vi "dvp Vi Set Target Format.vi"(10 "TargetFormat":u32(ring) items=["S_RAW8"=0, "S_RAW10"=1, "S_RAW12"=2, "S_RAW14"=3, "S_RAW16"=4, "S_BGR24"=10, "S_YCBCR_411"=20, "S_YCBCR_422"=21, "S_YCBCR_444"=22, "S_MONO8"=30, "S_MONO10"=31, "S_MONO12"=32, "S_MONO14"=33, "S_MONO16"=34], 11 "handle":u32) -> (3 "function return":u32(ring))   [LabVIEW 2018, in "LabViewDVPCamera.lvlib"]
doc: "LabviewDvp2Api dvpStatus dvpViSetTargetFormat(dvpHandle handle, dvpStreamFormat TargetFormat);"
uses:
  LabViewDVPCamera.lvlib
  LabViewDVPCamera/LabViewDVPCamera.dll
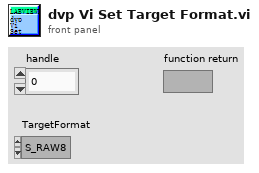
[diagram p1: front panel]
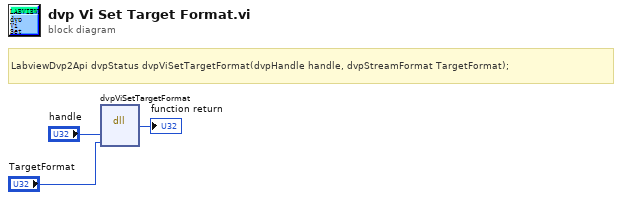
[diagram p0: block diagram]
diagram:
  # "LabviewDvp2Api dvpStatus dvpViSetTargetFormat(dvpHandle handle, dvpStreamFormat TargetFormat);"
  n1 = dll-call lib="C:/Program Files (x86)/DVP2 Labview cn 64/Sample/LabViewDVPCamera/LabViewDVPCamera.*" fn="dvpViSetTargetFormat"("handle"="handle", "TargetFormat"="TargetFormat") -> (→"function return":u32)  [unwired: 5 in, 2 out]
